vi "Project.vi"(8 "error in":errorcluster, 10 "sceneCoords in":T1, 11 "class data in":refnum<class "SceneRoot.lvclass">) -> (0 "error out":errorcluster, 2 "winCoords out":T2, 3 "class data out":refnum<class "SceneRoot.lvclass">)   [LabVIEW 2010, in "RenderBase.lvlib" / "SceneRoot.lvclass"]
doc: "Converts scene coordinates into window coordinates."
uses:
  SceneRoot.lvclass
  <vilib>/Utility/miscctls.llb/LVPoint32TypeDef.ctl
  <vilib>/Utility/miscctls.llb/LV3DPointTypeDef.ctl
  SceneRoot.lvclass/SceneRoot.ctl
  <vilib>/Analysis/baseanly.llb/Real A x B.vi
  <vilib>/Analysis/baseanly.llb/A x Vector.vi
  <vilib>/Analysis/NI_AALBase.lvlib
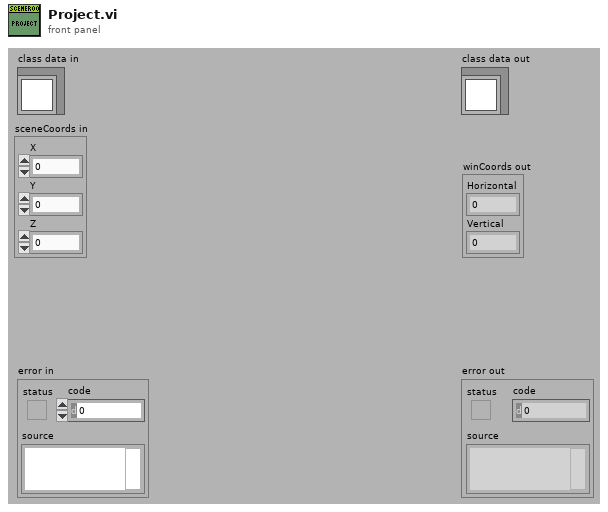
[diagram p1: front panel]
types:
  T1 = typedef "LV3DPointTypeDef.ctl" = cluster{"X":sgl, "Y":sgl, "Z":sgl}
  T2 = typedef "LVPoint32TypeDef.ctl" = cluster{"Horizontal":i32, "Vertical":i32}
  T3 = typedef "NI_Matrix.lvlib/RealMatrix.ctl" = dbl[][]
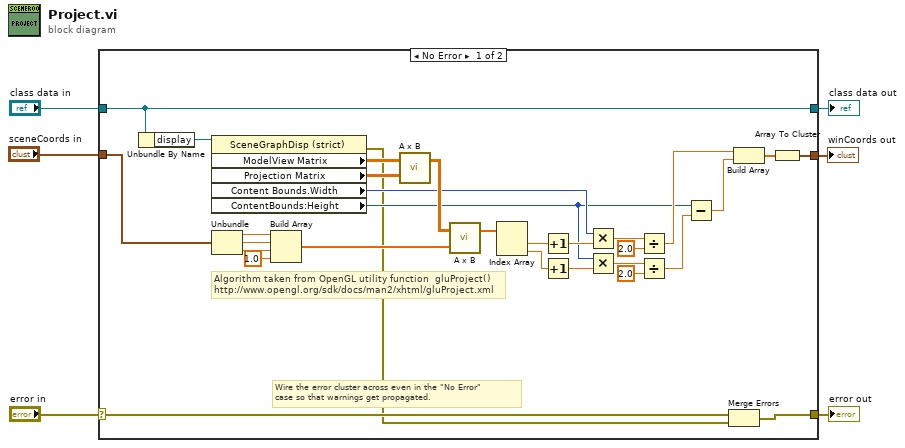
[diagram p0: block diagram]
diagram:
  n1 = case shown="No Error" "error in" {
    selector: "error in" -> [w9 w38]
    tunnel: [w8 w38] -> w5
    tunnel: [w36 w37] -> w3
    tunnel: "class data in" -> [w36 w37]
    tunnel: "sceneCoords in" -> [w11 _]
    tunnel: [w10 _] -> w1
    frame No Error {
      # "Algorithm taken from OpenGL utility function  gluProject()\nhttp://www.opengl.org/sdk/docs/man2/xhtml/gluProject.xml"
      # "Wire the error cluster across even in the \"No Error\"\ncase so that warnings get propagated."
      n2 = Unbundle By Name(w36) -> ("display"=w12:refnum<vi>)
      n3 = property class="SceneGraphDisp (strict)"(reference=w12) -> (error out=w7:errorcluster, "ModelView Matrix"=w34:sgl[][], "Projection Matrix"=w35:sgl[][], "Content Bounds.Width"=w20:u32, "ContentBounds:Height"=w13:u32)  [unwired: 1 in, 1 out]
      n4 = Unbundle(w11) -> ("X"=w29:sgl, "Y"=w28:sgl, "Z"=w27:sgl)
      n5 = Build Array(w29, w28, w27, sgl 1.0 ("element")) -> (w24:sgl[])
      n6 = call-poly <vilib>:"A x B.vi"("B"=w35, "A"=w34) -> ("A x B"=w25:T3)  [unwired: 1 out]
      n7 = call-poly <vilib>:"A x B.vi"("Vector"=w24, "A"=w25) -> ("A x Vector"=w33:dbl[])  [unwired: 1 out]
      n8 = Index Array(array=w33) -> (element #1=w32:dbl, element #2=w30:dbl)  [unwired: 2 in]
      n9 = Increment(x=w32) -> (x+1=w21:dbl)
      n10 = Increment(x=w30) -> (x+1=w22:dbl)
      n11 = Multiply(x=w20, y=w21) -> (x*y=w23:dbl)
      n12 = Multiply(x=w13, y=w22) -> (x*y=w18:dbl)
      n13 = Divide(x=w23, y=2.0) -> (x/y=w19:dbl)
      n14 = Divide(x=w18, y=2.0) -> (x/y=w15:dbl)
      n15 = Subtract(x=w13, y=w15) -> (x-y=w14:dbl)
      n16 = Merge Errors(w9, w7) -> (w8:errorcluster)
      n17 = Build Array(w19, w14) -> (w31:dbl[])
      n18 = Array To Cluster(array=w31) -> (cluster=w10:cluster{"[0]":dbl, "[1]":dbl})
    }
    frame Error {
    }
  }
  "error out" <- w5
  "class data out" <- w3
  "winCoords out" <- w1
